vi "Enable FP.vi"(7 "Ignore?":bool, 8 "error in (no error)":errorcluster, 11 "FP Controls in":refnum<class "FP Controls.lvclass">) -> (0 "error out":errorcluster, 3 "FP Controls out":refnum<class "FP Controls.lvclass">)   [LabVIEW 2012, in "Configuration Grandmaster.lvlib" / "FP Controls.lvclass"]
uses:
  FP Controls.lvclass
  FP Controls.lvclass/FP Controls.ctl
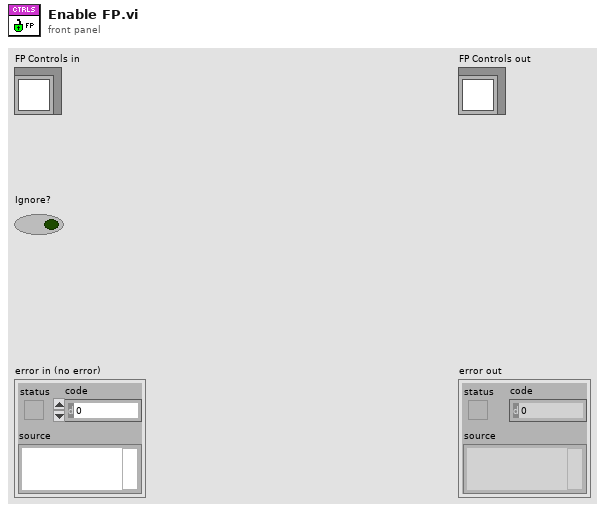
[diagram p1: front panel]
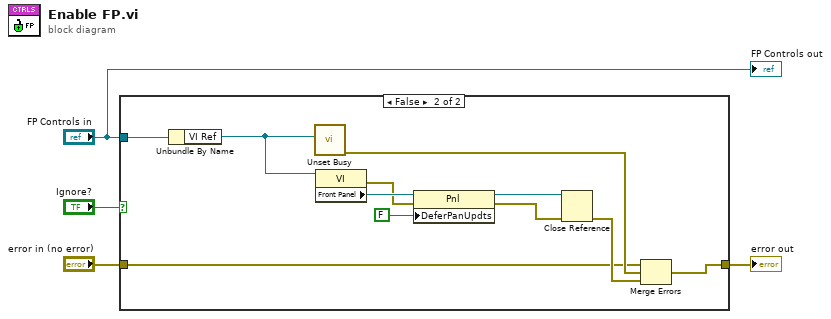
[diagram p0: block diagram]
diagram:
  n1 = case shown="False" "Ignore?" {
    tunnel: "FP Controls in" -> [_ w16]
    tunnel: "error in (no error)" -> [w5 w7]
    tunnel: [w5 w6] -> w2
    frame True {
    }
    frame False {
      n2 = Unbundle By Name(w16) -> ("VI Ref"=w10:refnum<vi>)
      n3 = call <vilib>:"Unset Busy.vi"("VI reference (current VI)"=w10) -> ("error out"=w9:errorcluster)  [unwired: 10 in]
      n4 = property class="VI"(reference=w10) -> (error out=w12:errorcluster, "Front Panel"=w15:refnum<vi>)  [unwired: 1 in, 1 out]
      n5 = property class="Pnl"(reference=w15, error in=w12, "DeferPanUpdts"=FALSE ("Defer Panel Updates")) -> (reference out=w14:refnum<vi>, error out=w13:errorcluster)
      n6 = Close Reference(reference=w14, error in (no error)=w13) -> (error out=w8:errorcluster)
      n7 = Merge Errors(w7, w9, w8) -> (w6:errorcluster)
    }
  }
  "error out" <- w2
  "FP Controls out" <- "FP Controls in"
